vi "_Construct Peak List.vi"(5 "Search Window":dbl=3.0 min=0.1 format="%#.6f", 6 "Peak List":T1[](array[typedef]), 7 "RefMass":dbl[](array[numeric])) -> (1 "Array":dbl[][](array[numeric]), 2 "# of Peaks":i32, 3 "Table":string[][](table))   [LabVIEW 2012]
uses:
  Type/_Peak Property.ctl
panel:
  # "Apex"
  # "Centroid"
  # "Baseline"
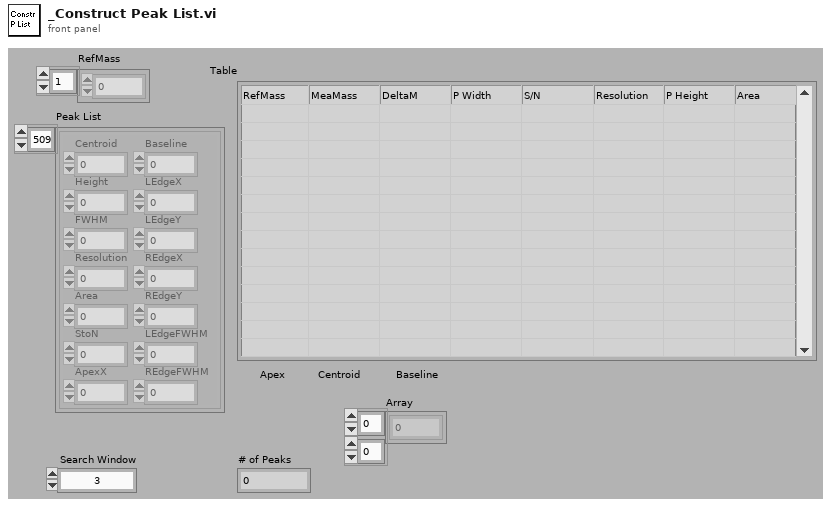
[diagram p1: front panel]
types:
  T1 = typedef "_Peak Property.ctl" = cluster{"Centroid":dbl, "Height":dbl, "FWHM":dbl, "Resolution":dbl, "Area":dbl, "StoN":dbl, "ApexX":dbl, "Baseline":dbl, "LEdgeX":dbl, "LEdgeY":dbl, "REdgeX":dbl, "REdgeY":dbl, "LEdgeFWHM":dbl, "REdgeFWHM":dbl}
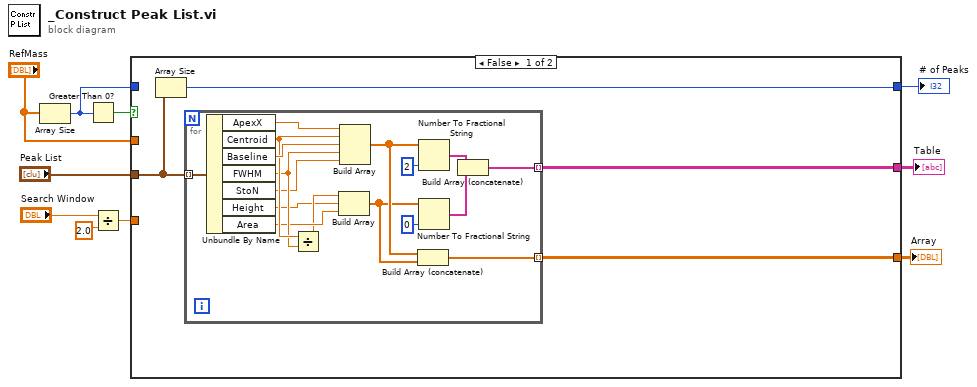
[diagram p0: block diagram]
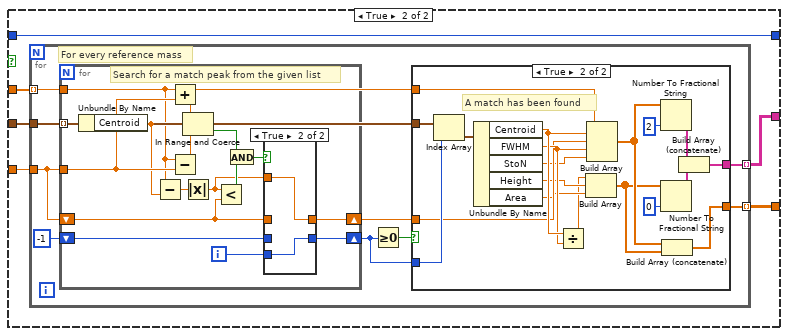
[diagram p2: hidden frame]
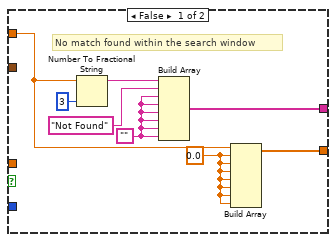
[diagram p3: hidden frame]
diagram:
  n1 = Array Size(array="RefMass") -> (size(s)=w9:i32)
  n2 = Greater Than 0?(x=w9) -> (x > 0?=w10:bool)
  n3 = Divide(x="Search Window", y=2.0) -> (x/y=w3:dbl)
  n4 = case shown="False" w10 {
    tunnel: w9 -> [_ w37]
    tunnel: [w14 w37] -> w8
    tunnel: "RefMass" -> [_ w36]
    tunnel: "Peak List" -> [w13 w35]
    tunnel: [w12 w33] -> w5
    tunnel: w3 -> [_ w34]
    tunnel: [w11 w32] -> w1
    frame False {
      n5 = Array Size(array=w13) -> (size(s)=w14:i32)
      n6 = for {
        tunnel: w13 -> [w31] mode=indexing
        tunnel: [w21] -> w12 mode=indexing
        tunnel: [w18] -> w11 mode=indexing
        n7 = Unbundle By Name(w31) -> ("ApexX"=w30:dbl, "Centroid"=w28:dbl, "Baseline"=w29:dbl, "FWHM"=w27:dbl, "StoN"=w17:dbl, "Height"=w15:dbl, "Area"=w22:dbl)
        n8 = Divide(x=w28, y=w27) -> (x/y=w16:dbl)
        n9 = Build Array(w16, w15, w22) -> (w19:dbl[])
        n10 = Build Array(w30, w28, w29, w27, w17) -> (w20:dbl[])
        n11 = Build Array (concatenate)(w20, w19) -> (w18:dbl[])
        n12 = Number To Fractional String(number=w20, precision (6)=i16 2) -> (F-format string=w25:string[])  [unwired: 2 out]
        n13 = Number To Fractional String(number=w19, precision (6)=i16 0) -> (F-format string=w24:string[])  [unwired: 2 out]
        n14 = Build Array (concatenate)(w25, w24) -> (w21:string[])
      }
    }
    frame True {
      n15 = for {
        tunnel: w36 -> [w44] mode=indexing
        tunnel: w35 -> [w42]
        tunnel: w34 -> [w39]
        tunnel: [w40] -> w33 mode=indexing
        tunnel: [w38] -> w32 mode=indexing
        # "For every reference mass"
        n16 = for {
          tunnel: w42 -> [w89] mode=indexing
          tunnel: w44 -> [w85]
          shift-right: [w78] -> w43
          shift-left: w39 -> [w79]
          tunnel: w39 -> [w86]
          shift-right: [w76] -> w41
          shift-left: -1 -> [w77]
          i -> [w74]
          # "Search for a match peak from the given list"
          n17 = Unbundle By Name(w89) -> ("Centroid"=w84:dbl)
          n18 = Subtract(x=w85, y=w84) -> (x-y=w83:dbl)
          n19 = Add(x=w85, y=w86) -> (x+y=w87:dbl)
          n20 = Subtract(x=w85, y=w86) -> (x-y=w88:dbl)
          n21 = In Range and Coerce(upper limit=w87, x=w84, lower limit=w88) -> (In Range?=w82:bool)  [unwired: 1 out]
          n22 = Absolute Value(x=w83) -> (abs(x)=w75:dbl)
          n23 = Less?(x=w75, y=w79) -> (x < y?=w81:bool)
          n24 = And(x=w82, y=w81) -> (x .and. y?=w80:bool)
          n25 = case shown="True" w80 {
            tunnel: [w91 w92] -> w78
            tunnel: w79 -> [w91 _]
            tunnel: [w90 w93] -> w76
            tunnel: w77 -> [w90 _]
            tunnel: w75 -> [_ w92]
            tunnel: w74 -> [_ w93]
            frame False {
            }
            frame True {
            }
          }
        }
        n26 = Greater Or Equal To 0?(x=w41) -> (x >= 0?=w45:bool)
        n27 = case shown="True" w45 {
          tunnel: w44 -> [w49 w69]
          tunnel: w43 -> [_ w68]
          tunnel: w42 -> [_ w73]
          tunnel: w41 -> [_ w72]
          tunnel: [w50 w62] -> w40
          tunnel: [w47 w58] -> w38
          frame False {
            w48 = 0.0 ("element")
            w51 = ""
            # "No match found within the search window"
            n28 = Number To Fractional String(number=w49, precision (6)=i16 3) -> (F-format string=w53:string)  [unwired: 2 out]
            n29 = Build Array(w53, "Not Found", w51, w51, w51, w51, w51, w51) -> (w50:string[])
            n30 = Build Array(w49, w48, w48, w48, w48, w48, w48, w48) -> (w47:dbl[])
          }
          frame True {
            # "A match has been found"
            n31 = Index Array(array=w73, index=w72) -> (element=w67:T1)
            n32 = Unbundle By Name(w67) -> ("Centroid"=w71:dbl, "FWHM"=w70:dbl, "StoN"=w57:dbl, "Height"=w56:dbl, "Area"=w65:dbl)
            n33 = Divide(x=w71, y=w70) -> (x/y=w55:dbl)
            n34 = Build Array(w55, w56, w65) -> (w59:dbl[])
            n35 = Build Array(w69, w71, w68, w70, w57) -> (w60:dbl[])
            n36 = Number To Fractional String(number=w60, precision (6)=i16 2) -> (F-format string=w64:string[])  [unwired: 2 out]
            n37 = Number To Fractional String(number=w59, precision (6)=i16 0) -> (F-format string=w63:string[])  [unwired: 2 out]
            n38 = Build Array (concatenate)(w60, w59) -> (w58:dbl[])
            n39 = Build Array (concatenate)(w64, w63) -> (w62:string[])
          }
        }
      }
    }
  }
  "# of Peaks" <- w8
  "Table" <- w5
  "Array" <- w1
